vi "check_user.vi"(10 "id":string, 11 "lc_num":string) -> (0 "error":errorcluster caption="error out 4", 2 "check":bool)   [LabVIEW 2017, in "Lib_code.lvlib"]
uses:
  Lib_code.lvlib
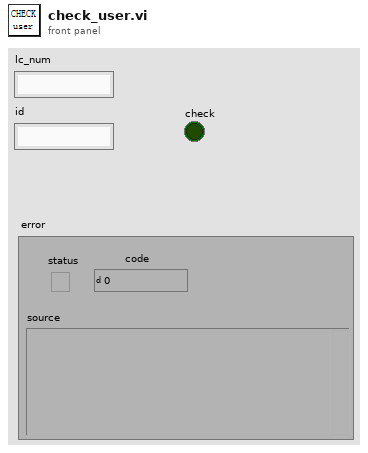
[diagram p1: front panel]
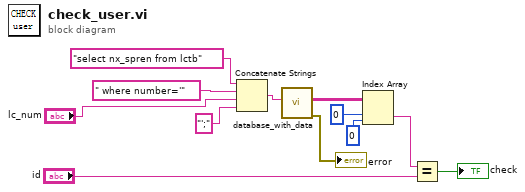
[diagram p0: block diagram]
diagram:
  n1 = Concatenate Strings("select nx_spren from lctb" ("Command Text"), " where number='" ("Command Text"), "lc_num", "';" ("字符串")) -> (w6:string)
  n2 = call "database_with_data.vi"("input"=w6) -> ("error"=→"error":errorcluster, "Data"=w4:string[][])  [unwired: 9 in]
  n3 = Index Array(array=w4, index (row)=0 ("索引 (行)"), index (col)=0 ("禁用的索引 (列)")) -> (element=w3:string)
  n4 = Equal?(x=w3, y="id") -> (x = y?=→"check":bool)
